vi "Hand_Store_Data.vi"(9 "Current load (mA)":dbl[](array[numeric]), 10 "Position (bits)":dbl[](array[numeric])) -> (2 "Motors info":T1(array[cluster]))   [LabVIEW 2015]
panel:
  in  "Motors info in":T1(array[cluster])=[{"Motor "="Wrist rotation", "Position (% Max position)"=0.0, "Current load (mA)"=0.0}, {"Motor "="Wrist adduction", "Position (% Max position)"=0.0, "Current load (mA)"=0.0}, {"Motor "="Wrist flexion", "Position (% Max position)"=0.0, "Current load (mA)"=0.0}, {"Motor "="Thumb adduction", "Position (% Max position)"=0.0, "Current load (mA)"=0.0}, {"Motor "="Thumb flexion", "Position (% Max position)"=0.0, "Current load (mA)"=0.0}, {"Motor "="Index flexion", "Position (% Max position)"=0.0, "Current load (mA)"=0.0}, {"Motor "="Middle fingers flexion", "Position (% Max position)"=0.0, "Current load (mA)"=0.0}]
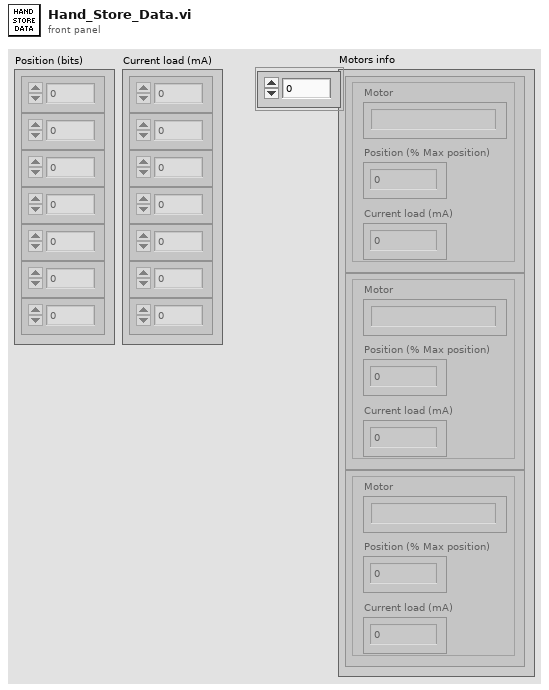
[diagram p1: front panel]
types:
  T1 = cluster{"Motor ":string, "Position (% Max position)":dbl, "Current load (mA)":dbl}[]
  T2 = cluster{"Motor ":string, "Position (% Max position)":dbl, "Current load (mA)":dbl}
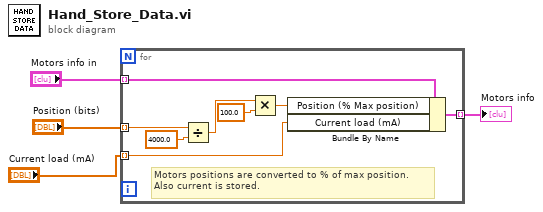
[diagram p0: block diagram]
diagram:
  n1 = for {
    tunnel: "Position (bits)" -> [w9] mode=indexing
    tunnel: "Motors info in" -> [w7] mode=indexing
    tunnel: [w6] -> w1 mode=indexing
    tunnel: "Current load (mA)" -> [w5] mode=indexing
    # "Motors positions are converted to % of max position.\nAlso current is stored."
    n2 = Divide(x=w9, y=4000.0) -> (x/y=w11:dbl)
    n3 = Multiply(x=w11, y=100.0) -> (x*y=w8:dbl)
    n4 = Bundle By Name(cluster=w7, "Position (% Max position)"=w8, "Current load (mA)"=w5) -> (w6:T2)
  }
  "Motors info" <- w1
